vi "Read Event Registration.vi"(10 "channel":T1) -> (2 "Event Registration Refnum":refnum<event-registration>)   [LabVIEW 2020, in "Event Messenger Priority.lvlib"]
doc: "<p>Reads an <a href=\"nihelplauncher://docs/csh?context=lvcore_lvconcepts_using_events_in_labview\">event registration</a> refnum for an Event Messenger Priority <a href=\"nihelplauncher://docs/csh?context=lvcore_lvconcepts_channel_wires_intro\">channel</a>.</p>"
uses:
  Event Messenger Priority.lvlib
  ChannelOp.ctl
  ))Channel.ctl
  Element.ctl
  Event Data.ctl
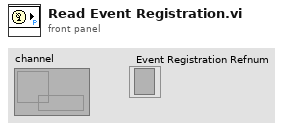
[diagram p1: front panel]
types:
  T1 = typedef "Event Messenger Priority.lvlib/))Channel.ctl" = refnum<queue>
  T2 = typedef "Event Messenger Priority.lvlib/ChannelOp.ctl" = enum16{"init", "write", "register", "replicate", "probe"}
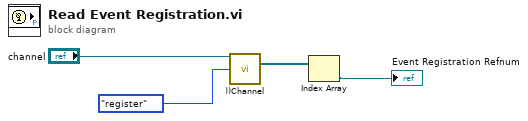
[diagram p0: block diagram]
diagram:
  n1 = call "))Channel.vi"("channel out"="channel", "channelOp"=ChannelOp."register") -> ("Event Registration Refnum"=w3:refnum<event-registration>[])  [unwired: 9 in, 4 out]
  n2 = Index Array(array=w3) -> (element=→"Event Registration Refnum":refnum<event-registration>)  [unwired: 1 in]
